vi "Set String.vi"(5 "use temporary file? (F)":bool, 8 "error in":errorcluster, 9 "value":string, 10 "variable name":string, 11 "GOLPI ref. in":T1={"pipe handle"={"lv_proc.dll file path"=path "", "process instance handle"=[], "debug mode"=FALSE, "debug data"=[]}, "fast read timeout [ms]"=500, "fast read settle time [ms]"=10, "fast read to multiple [ms]"=1, "max elements per input line"=100, "slow read timeout [ms]"=5000, "stdin double format specifier"="%_16e", "max elements per stdout output column"=100, "console mode bitstream"=FALSE, "bitstream first read timeout [ms]"=1000, "bitstream read timeout [ms]"=50, "struct transfer possible"=FALSE, "matlab mode"=FALSE}) -> (0 "error out":errorcluster, 3 "GOLPI ref. out":T1={"pipe handle"={"lv_proc.dll file path"=path "", "process instance handle"=[], "debug mode"=FALSE, "debug data"=[]}, "fast read timeout [ms]"=500, "fast read settle time [ms]"=10, "fast read to multiple [ms]"=1, "max elements per input line"=100, "slow read timeout [ms]"=5000, "stdin double format specifier"="%_16e", "max elements per stdout output column"=100, "console mode bitstream"=FALSE, "bitstream first read timeout [ms]"=1000, "bitstream read timeout [ms]"=50, "struct transfer possible"=FALSE, "matlab mode"=FALSE})   [LabVIEW 2020, in "GOLPI library.lvlib"]
doc: "Part of polymorph Set Variable.vi"
uses:
  GOLPI library.lvlib
  GOLPI reference Type Def.ctl
  Pipe Handle.ctl
  LV Process library.lvlib
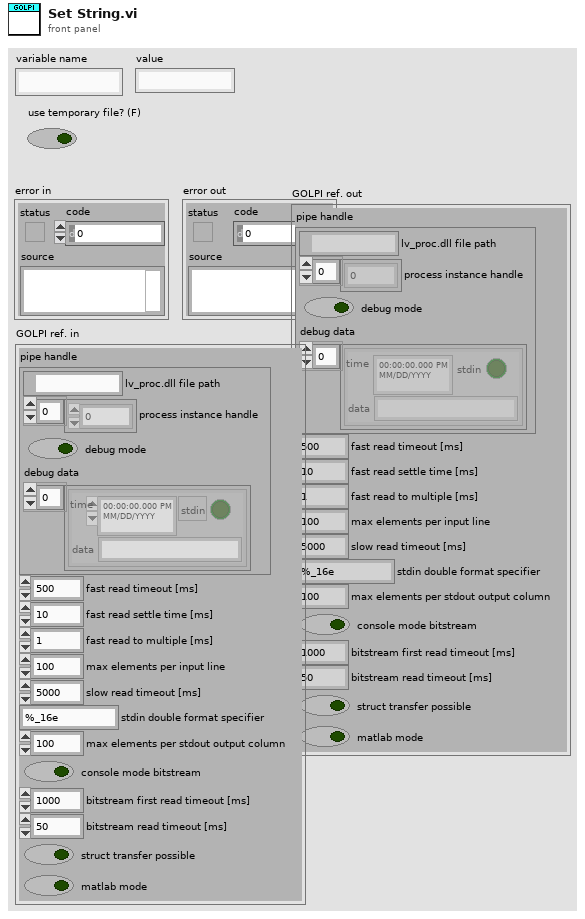
[diagram p1: front panel]
types:
  T1 = typedef "GOLPI library.lvlib/GOLPI reference Type Def.ctl" = cluster{"pipe handle":T2, "fast read timeout [ms]":u32, "fast read settle time [ms]":u32, "fast read to multiple [ms]":u32, "max elements per input line":u32, "slow read timeout [ms]":u32, "stdin double format specifier":string, "max elements per stdout output column":u32, "console mode bitstream":bool, "bitstream first read timeout [ms]":u32, "bitstream read timeout [ms]":u32, "struct transfer possible":bool, "matlab mode":bool}
  T2 = typedef "LV Process library.lvlib/Pipe Handle.ctl" = cluster{"lv_proc.dll file path":path, "process instance handle":u32[], "debug mode":bool, "debug data":cluster{"time":timestamp, "stdin":bool, "data":string}[]}
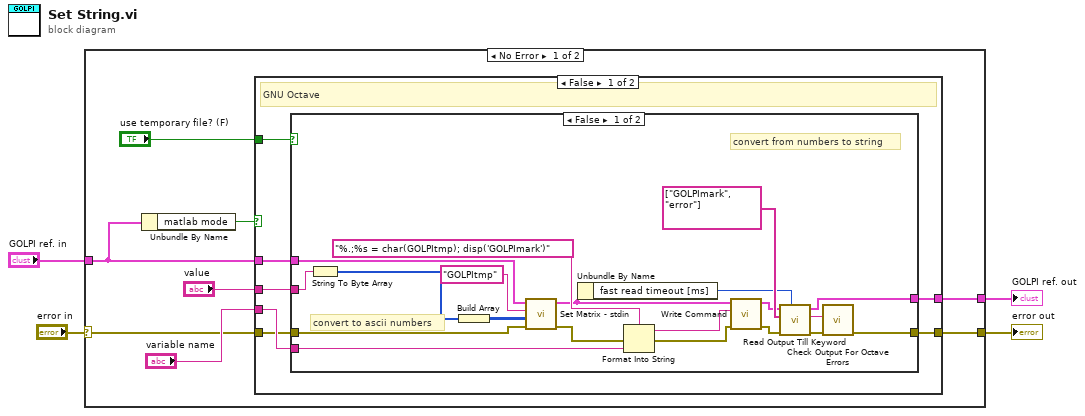
[diagram p0: block diagram]
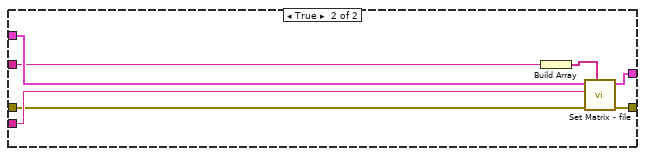
[diagram p2: hidden frame]
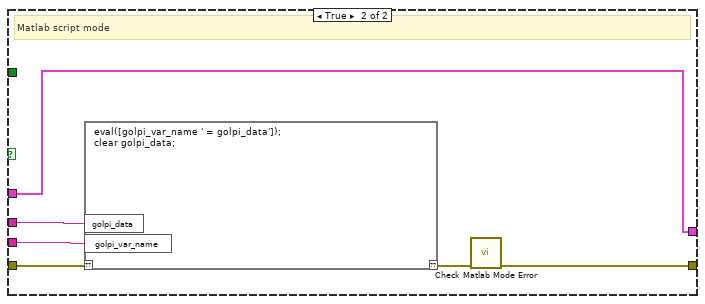
[diagram p3: hidden frame]
diagram:
  n1 = case shown="No Error" "error in" {
    selector: "error in" -> [w8 w54]
    tunnel: [w12 w54] -> w4
    tunnel: "GOLPI ref. in" -> [w6 w53]
    tunnel: [w11 w53] -> w1
    frame No Error {
      n2 = Unbundle By Name(w6) -> ("matlab mode"=w5:bool)
      n3 = case shown="False" w5 {
        tunnel: [w19 w47] -> w12
        tunnel: [w18 w51] -> w11
        tunnel: "variable name" -> [w17 w49]
        tunnel: "value" -> [w16 w50]
        tunnel: w8 -> [w15 w52]
        tunnel: w6 -> [w14 w51]
        tunnel: "use temporary file? (F)" -> [w13 _]
        frame False {
          # "GNU Octave"
          n4 = case shown="False" w13 {
            tunnel: [w39 w43] -> w19
            tunnel: [w38 w42] -> w18
            tunnel: w17 -> [w36 w46]
            tunnel: w16 -> [w26 w41]
            tunnel: w15 -> [w23 w44]
            tunnel: w14 -> [w22 w45]
            frame False {
              # "convert from numbers to string"
              # "convert to ascii numbers"
              n5 = String To Byte Array(string=w26) -> (unsigned byte array=w27:u8[])
              n6 = Build Array(w27) -> (w25:u8[][])
              n7 = call "Set Matrix - stdin.vi"("error in"=w23, "value"=w25, "variable name"="GOLPItmp", "GOLPI ref. in"=w22) -> ("error out"=w21:errorcluster, "GOLPI ref. out"=w20:T1)  [unwired: 6 in]
              n8 = Unbundle By Name(w20) -> ("fast read timeout [ms]"=w28:u32)
              n9 = Format Into String(format string="%.;%s = char(GOLPItmp); disp('GOLPImark')", error in=w21, w36) -> (resulting string=w34:string, error out=w35:errorcluster)  [unwired: 1 in]
              n10 = call "Write Command.vi"("error in"=w35, "command"=w34, "GOLPI ref. in"=w20) -> ("error out"=w33:errorcluster, "GOLPI ref. out"=w30:T1)  [unwired: 7 in]
              n11 = call "Read Output Till Keyword.vi"("timeout [ms]"=w28, "error in"=w33, "keywords"=string[] ["GOLPImark", "error"], "GOLPI ref. in"=w30) -> ("error out"=w32:errorcluster, "read buffer"=w29:string, "GOLPI ref. out"=w38:T1)  [unwired: 4 in, 1 out]
              n12 = call "Check Output For Octave Errors.vi"("error in"=w32, "read buffer"=w29) -> ("error out"=w39:errorcluster)  [unwired: 9 in]
            }
            frame True {
              n13 = Build Array(w41) -> (w40:string[])
              n14 = call "Set Matrix - file.vi"("string array"=w40, "error in (no error)"=w44, "variable name"=w46, "GOLPI ref. in"=w45) -> ("error out"=w43:errorcluster, "GOLPI ref. out"=w42:T1)  [unwired: 6 in]
            }
          }
        }
        frame True {
          # "Matlab script mode"
          n15 = script code="eval([golpi_var_name ' = golpi_data']);\nclear golpi_data;"("??"=w52, "golpi_var_name"=w49, "golpi_data"=w50) -> ("??"=w48:errorcluster)
          n16 = call "Check Matlab Mode Error.vi"("error in"=w48) -> ("error out"=w47:errorcluster)  [unwired: 10 in]
        }
      }
    }
    frame Error {
    }
  }
  "error out" <- w4
  "GOLPI ref. out" <- w1
